vi "AMZ_S3_APIHLP_Convert LoggingPermission String to Enum.vi"(4 "LoggingPermission String":string) -> (1 "Permission":T1)   [LabVIEW 2015, in "LV Interface for Amazon S3.lvlib"]
doc: "Convert the Storage Class represented as a String to the Enum typedef representation."
uses:
  LV Interface for Amazon S3.lvlib
  Typedefs/AMZ_S3_LoggingPermission.ctl
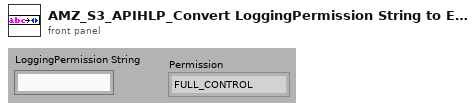
[diagram p1: front panel]
types:
  T1 = typedef "LV Interface for Amazon S3.lvlib/AMZ_S3_LoggingPermission.ctl" = enum16{"FULL_CONTROL", "READ", "WRITE"}
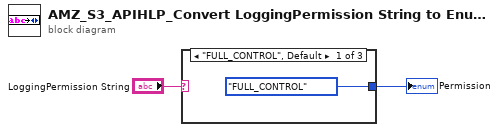
[diagram p0: block diagram]
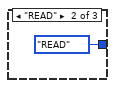
[diagram p2: hidden frame]
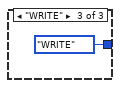
[diagram p3: hidden frame]
diagram:
  n1 = case shown="\"FULL_CONTROL\", Default" "LoggingPermission String" {
    tunnel: [AMZ_S3_LoggingPermission."FULL_CONTROL" ("Permission") AMZ_S3_LoggingPermission."READ" ("Permission") AMZ_S3_LoggingPermission."WRITE" ("Permission")] -> w1
    frame "FULL_CONTROL", Default {
    }
    frame "READ" {
    }
    frame "WRITE" {
    }
  }
  "Permission" <- w1
